vi "HapticSPM_force_two-state.vi"() -> ()   [LabVIEW 2023]
uses:
  Haptic-Programming-Interface/LabVIEW VIs/Haptic Prog Interface/Haptic Prog Interface.lvlib
panel:
  out "k":dbl format="%#_13g"
  out "Setpoint":dbl format="%#_13g"
  out "Energy Level (Dynamic)":picture
  out "Energy Level (Static)":picture
  out "Force Function":string
  in  "Input Function":i32 min=0 max=2 step=1
  out "Potential vs Distance":cluster{dbl[], dbl[]}(graph)
  out "Force vs Distance":cluster{dbl[], dbl[]}(graph)
  out "Z-Position (pm)":dbl caption="Numeric" min=0.0 format="%#.1p"
  out "Force":dbl(knob) scale=-3.0..3.0
  in  "Gain":dbl=1.0 caption="Numeric" format="%.1g"
  # "Super Ultra Mega Haptic SPM Controller 3000"
  # "Height"
  # "Move pen in all three dimensions to calibrate before feeling surface\n\nClick \"ENTER\" to turn off recommended settings\n\nChange \"Setpoint\" and \"k\" parameters to adjust the feel of the force\n\nUse the \"PAGE UP\" or \"PAGE DOWN\" key to change the force function\n\nHold the pen as high as possible before changing force functions"
  # "Force"
  # "create new version with the feynman book stuff\n\nensure that the line of reasoning is physically accurate\n\ncreate bonding picture on this mode"
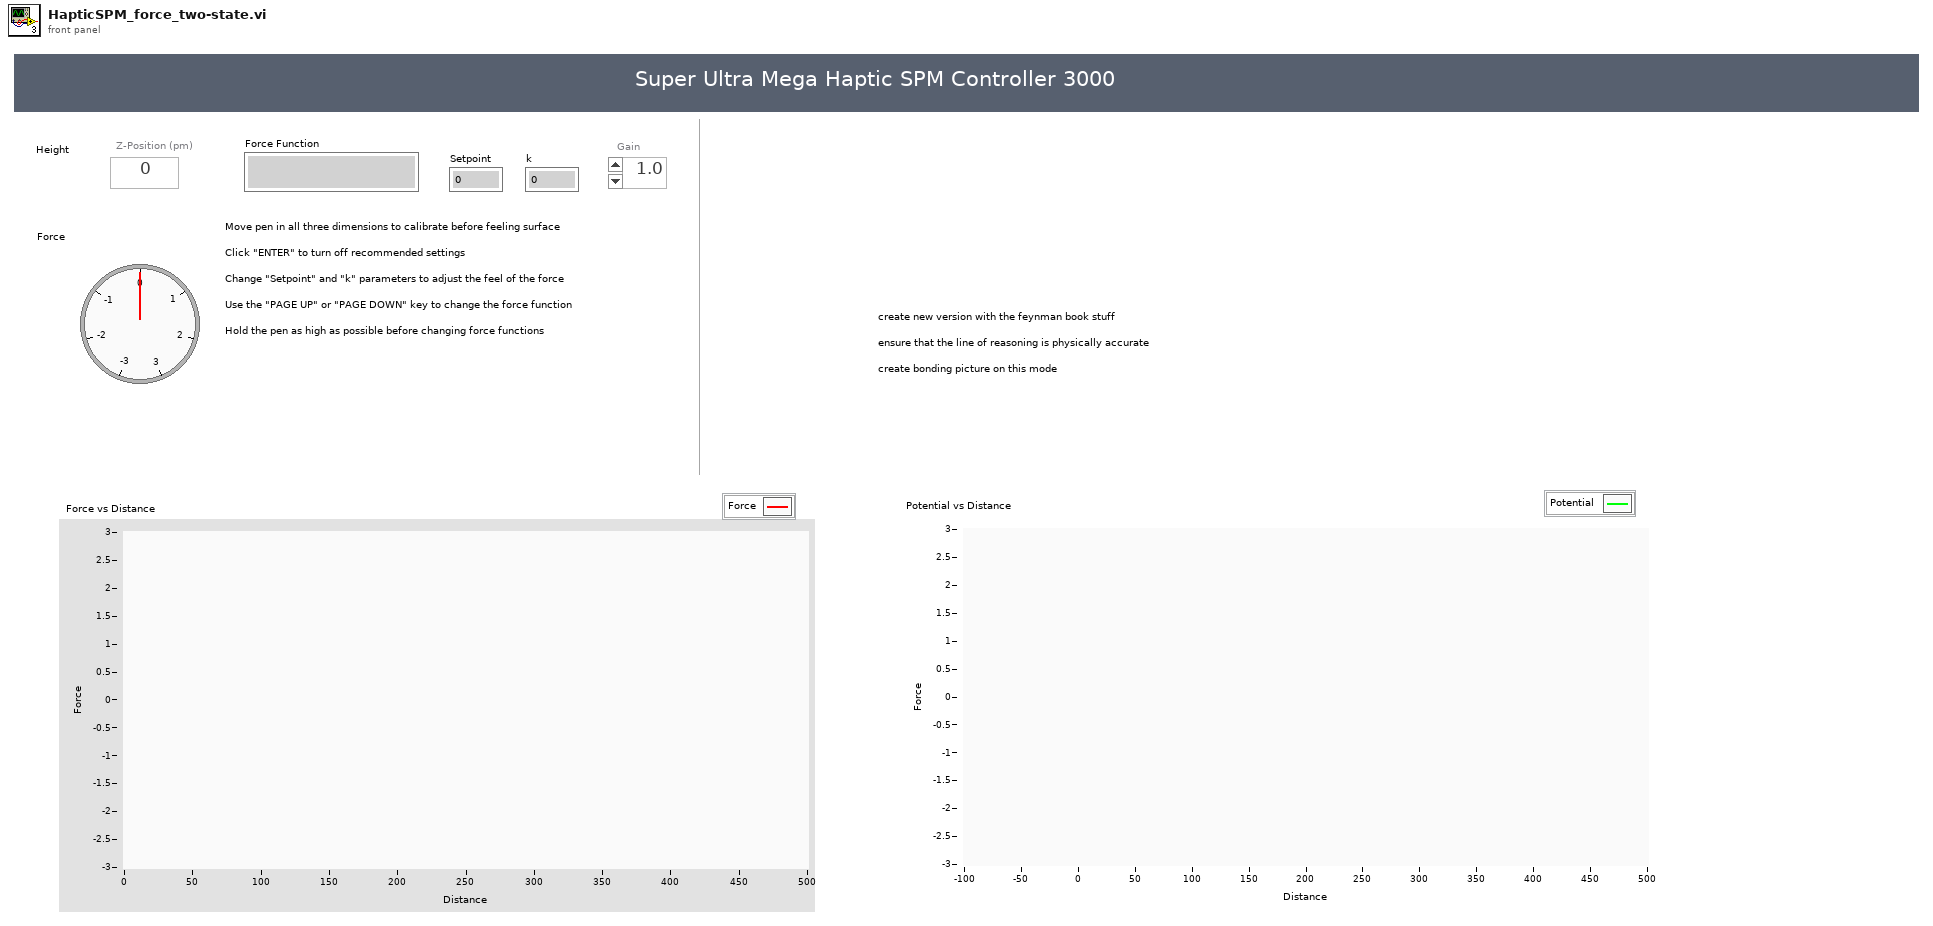
[diagram p1: front panel]
types:
  T1 = cluster{"Fx (N)":dbl, "Fy (N)":dbl, "Fz (N)":dbl}
  T2 = cluster{"kx (N/m)":dbl, "ky (N/m)":dbl, "kz (N/m)":dbl}
  T3 = cluster{"X Drag":bool, "Y Drag":bool, "Z Drag":bool}
  T4 = cluster{"x (mm)":dbl, "y (mm)":dbl, "z (mm)":dbl}
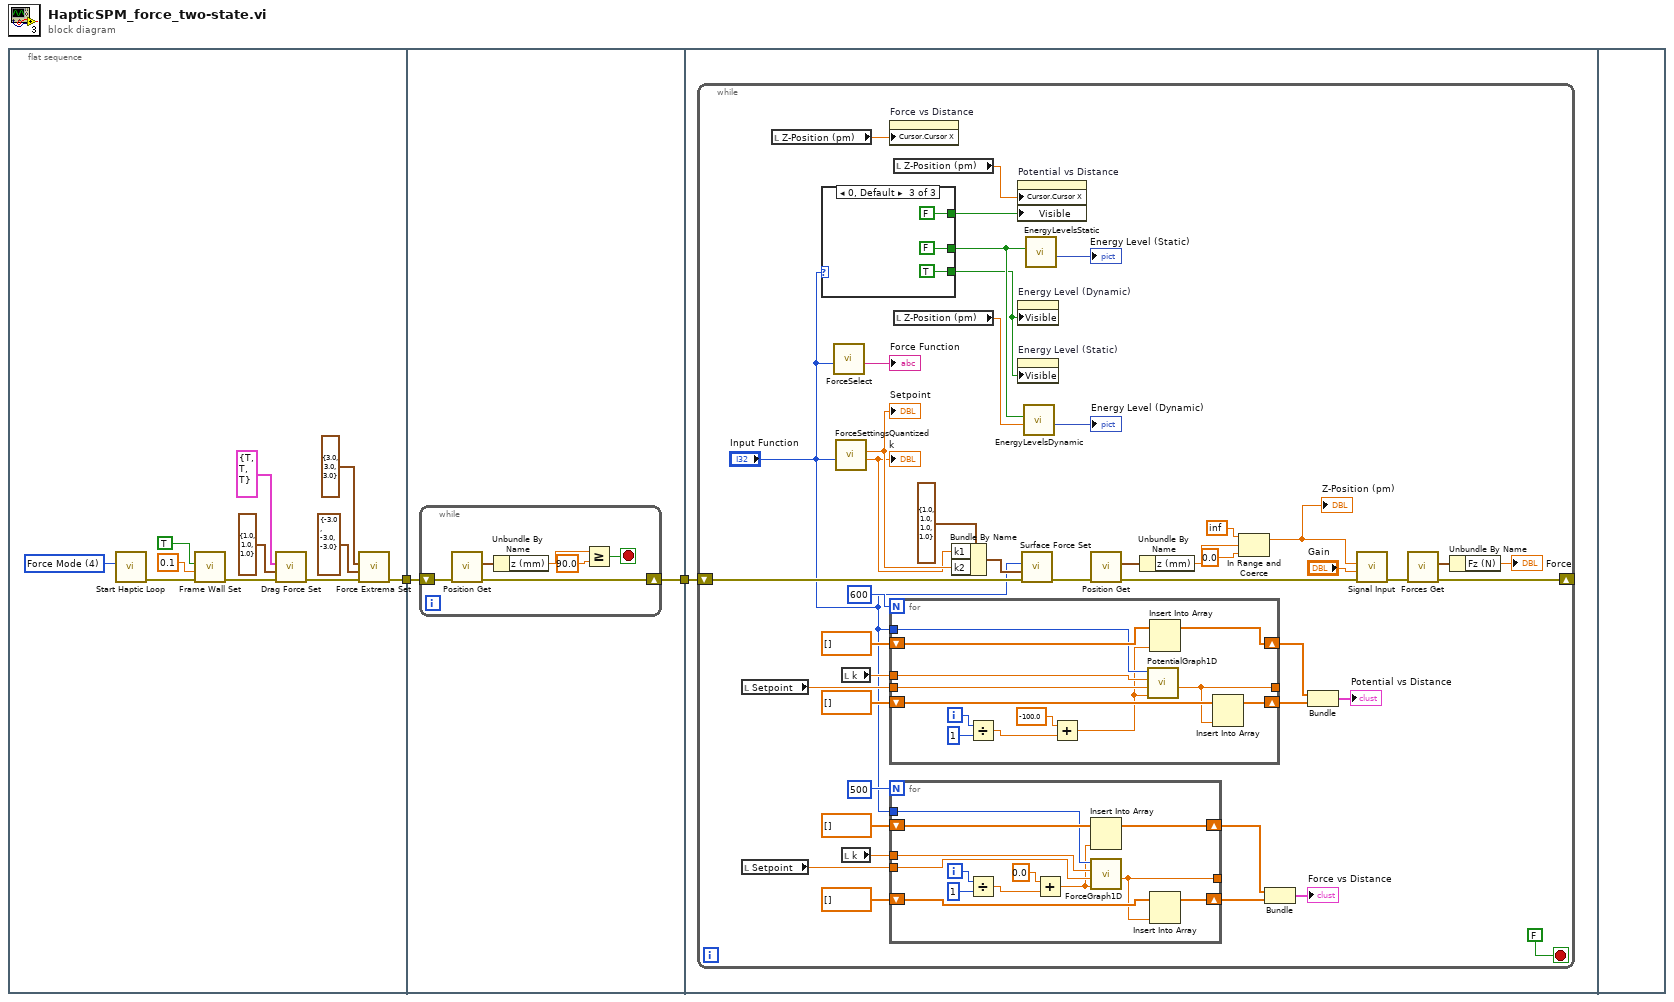
[diagram p0: block diagram]
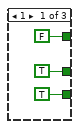
[diagram p2: hidden frame]
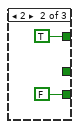
[diagram p3: hidden frame]
diagram:
  n1 = flat-sequence {
    tunnel: [w11] -> w2
    tunnel: w2 -> [w15]
    tunnel: [w14] -> w1
    tunnel: w1 -> [w22]
    frame #0 {
      w13 = u16 4 items=["Custom Mode", "Read Mode", "Write Mode", "Position Mode", "Force Mode"] ("Mode Selection")
      n2 = call "Start Haptic Loop.vi"("Mode Selection"=w13) -> ("error out"=w4:errorcluster)  [unwired: 10 in]
      n3 = call "Frame Wall Set.vi"("error in (no error)"=w4, "Wall Stiffness (N/m)"=0.1 ("Wall Stiffness"), "Restrict to Frame"=TRUE) -> ("error out"=w3:errorcluster)  [unwired: 8 in]
      n4 = call "Drag Force Set.vi"("error in (no error)"=w3, "Drag Coefficients (N/m)"=T2 {"kx (N/m)"=1.0, "ky (N/m)"=1.0, "kz (N/m)"=1.0} ("Drag Coefficients"), "Drag Force Toggles"=T3 {"X Drag"=TRUE, "Y Drag"=TRUE, "Z Drag"=TRUE}) -> ("error out"=w12:errorcluster)  [unwired: 8 in]
      n5 = call "Force Extrema Set.vi"("error in (no error)"=w12, "Minimum Force (N)"=T1 {"Fx (N)"=-3.0, "Fy (N)"=-3.0, "Fz (N)"=-3.0} ("Minimum Force"), "Maximum Force (N)"=T1 {"Fx (N)"=3.0, "Fy (N)"=3.0, "Fz (N)"=3.0} ("Maximum Force")) -> ("error out"=w11:errorcluster)  [unwired: 8 in]
    }
    frame #1 {
      n6 = while {
        shift-right: [w20] -> w14
        shift-left: w15 -> [w21]
        stop <- w16 stop-if-true
        n7 = call "Position Get.vi"("error in (no error)"=w21) -> ("error out"=w20:errorcluster, "Position"=w19:T4)  [unwired: 9 in]
        n8 = Unbundle By Name(w19) -> ("z (mm)"=w18:dbl)
        n9 = Greater Or Equal?(x=w18, y=90.0) -> (x >= y?=w16:bool)
      }
    }
    frame #2 {
      n10 = while {
        shift-right: [w50] -> _
        shift-left: w22 -> [w66]
        stop <- FALSE ("Boolean") stop-if-true
        n11 = local read "Setpoint"() -> (w41:dbl)
        n12 = local read "Setpoint"() -> (w52:dbl)
        n13 = local read "Z-Position (pm)"() -> (w51:dbl)
        n14 = case shown="0, Default" "Input Function" {
          tunnel: [FALSE TRUE FALSE] -> w39
          tunnel: [TRUE _ FALSE] -> w24
          tunnel: [TRUE FALSE TRUE] -> w23
          frame 1 {
          }
          frame 2 {
          }
          frame 0, Default {
          }
        }
        n15 = call "ForceSelect.vi"("Input Function"="Input Function") -> ("Force Function"=→"Force Function":string)  [unwired: 10 in]
        n16 = call "ForceSettingsQuantized.vi"("Function"="Input Function") -> ("k"=w25:dbl, "Setpoint"=w26:dbl)  [unwired: 9 in]
        "Setpoint" <- w26
        "k" <- w25
        n17 = local read "k"() -> (w42:dbl)
        n18 = local read "k"() -> (w53:dbl)
        n19 = property on="Force vs Distance" class="XYGraph (strict)"("Cursor.Cursor X"=w51) -> ()  [unwired: 2 in, 2 out]
        n20 = for {
          N: 600 -> [_]
          shift-right: [w87] -> w47
          shift-left: dbl[] [] -> [w85]
          shift-right: [w86] -> w48
          shift-left: dbl[] [] -> [w84]
          tunnel: "Input Function" -> [w80]
          tunnel: [w83] -> _
          tunnel: w41 -> [w82]
          tunnel: w42 -> [w81]
          i -> [w78]
          n21 = Divide(x=w78, y=1) -> (x/y=w77:dbl)
          n22 = Add(x=-100.0, y=w77) -> (x+y=w75:dbl)
          n23 = call "PotentialGraph1D.vi"("number"=w75, "Setpoint"=w82, "k"=w81, "Function"=w80) -> ("potential"=w83:dbl)  [unwired: 7 in]
          n24 = Insert Into Array(array=w84, new element=w75) -> (w86:dbl[])  [unwired: 1 in]
          n25 = Insert Into Array(array=w85, new element=w83) -> (w87:dbl[])  [unwired: 1 in]
        }
        n26 = for {
          N: 500 -> [_]
          shift-right: [w100] -> w58
          shift-left: dbl[] [] -> [w98]
          shift-right: [w99] -> w59
          shift-left: dbl[] [] -> [w97]
          tunnel: "Input Function" -> [w93]
          tunnel: [w96] -> _
          tunnel: w52 -> [w95]
          tunnel: w53 -> [w94]
          i -> [w91]
          n27 = Divide(x=w91, y=1) -> (x/y=w90:dbl)
          n28 = Add(x=0.0, y=w90) -> (x+y=w88:dbl)
          n29 = Insert Into Array(array=w97, new element=w88) -> (w99:dbl[])  [unwired: 1 in]
          n30 = call "ForceGraph1D.vi"("number"=w88, "Setpoint"=w95, "k"=w94, "Function"=w93) -> ("force"=w96:dbl)  [unwired: 7 in]
          n31 = Insert Into Array(array=w98, new element=w96) -> (w100:dbl[])  [unwired: 1 in]
        }
        n32 = local read "Z-Position (pm)"() -> (w40:dbl)
        n33 = local read "Z-Position (pm)"() -> (w27:dbl)
        n34 = Bundle By Name(cluster=cluster{"k1":dbl, "k2":dbl, "k3":dbl, "k4":dbl} {"k1"=1.0, "k2"=1.0, "k3"=1.0, "k4"=1.0} ("Force Constants"), "k1"=w25, "k2"=w26) -> (w62:cluster{"k1":dbl, "k2":dbl, "k3":dbl, "k4":dbl})
        n35 = property on="Potential vs Distance" class="XYGraph (strict)"("Cursor.Cursor X"=w40, "Visible"=w39) -> ()  [unwired: 2 in, 2 out]
        n36 = property on="Energy Level (Dynamic)" class="Pict"("Visible"=w23) -> ()  [unwired: 2 in, 2 out]
        n37 = property on="Energy Level (Static)" class="Pict"("Visible"=w23) -> ()  [unwired: 2 in, 2 out]
        n38 = call "Surface Force Set.vi"("error in (no error)"=w66, "Force Constants"=w62, "Force Settings"="Input Function") -> ("error out"=w36:errorcluster)  [unwired: 8 in]
        n39 = call "EnergyLevelsDynamic.vi"("Z-Position"=w27, "Up/Down Control"=w24) -> ("Energy Level"=→"Energy Level (Dynamic)":picture)  [unwired: 9 in]
        n40 = call "EnergyLevelsStatic.vi"("Up/Down Control"=w24) -> ("Energy Level"=→"Energy Level (Static)":picture)  [unwired: 10 in]
        n41 = call "Position Get.vi"("error in (no error)"=w36) -> ("error out"=w35:errorcluster, "Position"=w34:T4)  [unwired: 9 in]
        n42 = Unbundle By Name(w34) -> ("z (mm)"=w33:dbl)
        n43 = In Range and Coerce(upper limit=inf, x=w33, lower limit=0.0) -> (coerced(x)=w31:dbl)  [unwired: 1 out]
        "Z-Position (pm)" <- w31
        n44 = Bundle(w59, w58) -> (→"Force vs Distance":cluster{dbl[], dbl[]})  [unwired: 1 in]
        n45 = Bundle(w48, w47) -> (→"Potential vs Distance":cluster{dbl[], dbl[]})  [unwired: 1 in]
        n46 = call "Signal Input.vi"("error in (no error)"=w35, "Gain"="Gain", "Signal"=w31) -> ("error out"=w65:errorcluster)  [unwired: 8 in]
        n47 = call "Forces Get.vi"("error in (no error)"=w65) -> ("error out"=w50:errorcluster, "Force (N)"=w61:T1)  [unwired: 9 in]
        n48 = Unbundle By Name(w61) -> ("Fz (N)"=→"Force":dbl)
      }
    }
    frame #3 {
    }
  }
